vi "flashV5.vi"(6 "Register_Base_Address":u32=512 format="%x", 7 "flash_base_address":u32 format="%.0x", 8 "error in (no error)":errorcluster, 9 "empty":string, 10 "address":string="192.168.10.23", 11 "connection ID":refnum<k16>) -> (0 "error out":errorcluster, 1 "String":string, 2 "Out 2":u8 format="%.0x", 3 "connection ID 2":refnum<k16>)   [LabVIEW 2017]
panel:
  out "Array":i32[](array[numeric])
  out "data out 2":string
  out "String 2":string
  out "Out":u8 format="%.0x"
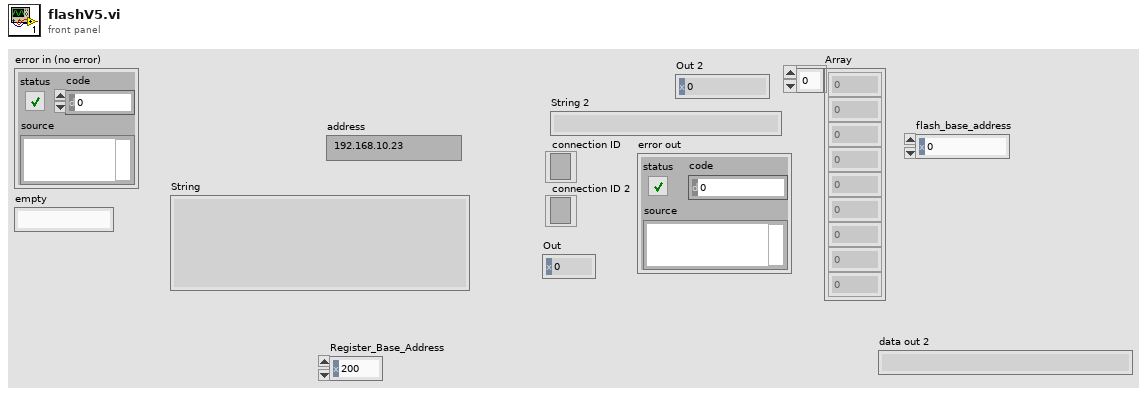
[diagram p1: front panel]
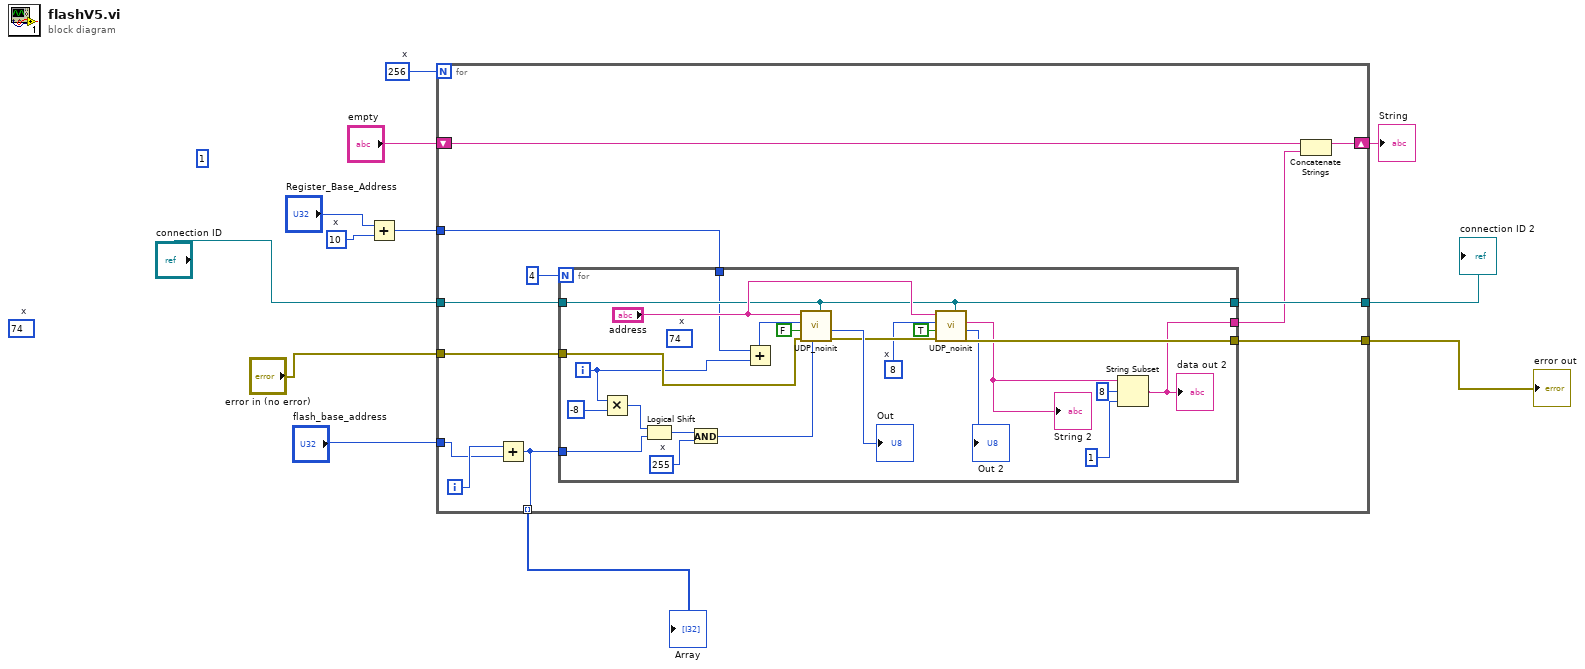
[diagram p0: block diagram]
diagram:
  w2 = u16 10  # x
  w10 = u16 256  # x
  (unwired) 1
  (unwired) u16 74  # x
  n1 = Add(x="Register_Base_Address", y=w2) -> (x+y=w1:u32)
  n2 = for {
    N: w10 -> [_]
    tunnel: "connection ID" -> [w23]
    tunnel: [w22] -> w11
    tunnel: [w21] -> w7
    shift-right: [w20] -> w8
    shift-left: "empty" -> [w19]
    tunnel: "error in (no error)" -> [w17]
    tunnel: "flash_base_address" -> [w15]
    tunnel: [w14] -> w4 mode=indexing
    tunnel: w1 -> [w13]
    i -> [w16]
    n3 = Add(x=w16, y=w15) -> (x+y=w14:u32)
    n4 = for {
      N: 4 -> [_]
      tunnel: w23 -> [w38]
      tunnel: [w38] -> w22
      tunnel: [w37] -> w21
      tunnel: [w30] -> w18
      tunnel: w17 -> [w33]
      tunnel: w14 -> [w28]
      tunnel: w13 -> [w25]
      i -> [w26]
      w36 = u16 8  # x
      w43 = u16 255  # x
      (unwired) u16 74  # x
      n5 = Multiply(x=w26, y=i16 -8) -> (x*y=w41:i32)
      n6 = Logical Shift(y=w41, x=w28) -> (x << y=w44:u32)
      n7 = And(x=w44, y=w43) -> (x .and. y?=w42:u32)
      n8 = Add(x=w25, y=w26) -> (x+y=w45:u32)
      n9 = call "UDP_noinit.vi"("connection ID"=w38, "In"=w42, "error in (no error)"=w33, "Read (TRUE)"=FALSE, "Address"=w45, "IP address"="address") -> ("error out"=w39:errorcluster, "Out"=→"Out":u8)  [unwired: 2 in, 1 out]
      n10 = call "UDP_noinit.vi"("connection ID"=w38, "error in (no error)"=w39, "Read (TRUE)"=TRUE, "Address"=w36, "IP address"="address") -> ("error out"=w37:errorcluster, "Out"=→"Out 2":u8, "received string"=w31:string)  [unwired: 3 in]
      "String 2" <- w31
      n11 = String Subset(string=w31, offset (0)=8, length (rest)=1 ("length (rest)")) -> (substring=w30:string)
      "data out 2" <- w30
    }
    n12 = Concatenate Strings(w19, w18) -> (w20:string)
  }
  "String" <- w8
  "connection ID 2" <- w11
  "error out" <- w7
  "Array" <- w4
